vi "PathPlanner_PathConstraints_FromJSON.vi"(11 "JSON String":string) -> (0 "Exists":bool, 3 "PathPlannerConstraints":T1={"MaxVelocityMps;"=0.0, "MaxAccelerationMpsSq;"=0.0, "MaxAngularVelRadPsEc;"=0.0, "MaxAngularAccRadPSecSq"=0.0, "Exists"=FALSE, "Unlimited"=FALSE, "NominalVoltageVolts"=12.0})   [LabVIEW 2019, in "PathPlanner24.lvlib"]
doc: "Create a path constraints object from json string\n \nInputs: \n - JSON String - string - string potentially containing a path constraints definition\n\nOutputs:\n - PathConstraint - cluster - The path constraints defined by the given json\n - Exists - boolean - TRUE if the string contained a path constraints definition"
uses:
  PathPlanner24.lvlib
  TypeDef/PathPlannerPathConstraints.ctl
  <vilib>/Rock Robotics/WPI/ThirdParty/JAS_Junk/TrajLib/Trajectory_Library.lvlib
panel:
  in  "globalConstraints":T2
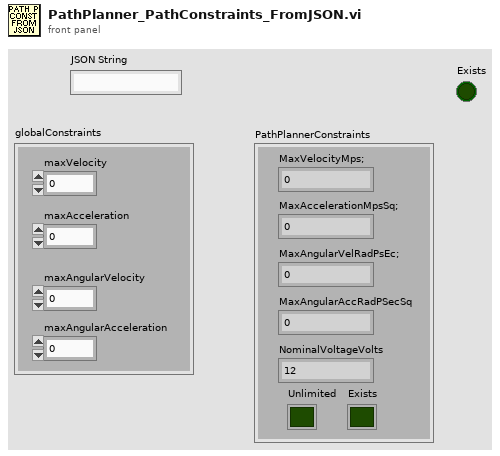
[diagram p1: front panel]
types:
  T1 = typedef "PathPlanner24.lvlib/PathPlannerPathConstraints.ctl" = cluster{"MaxVelocityMps;":dbl, "MaxAccelerationMpsSq;":dbl, "MaxAngularVelRadPsEc;":dbl, "MaxAngularAccRadPSecSq":dbl, "Exists":bool, "Unlimited":bool, "NominalVoltageVolts":dbl}
  T2 = cluster{"maxVelocity":dbl, "maxAcceleration":dbl, "maxAngularVelocity":dbl, "maxAngularAcceleration":dbl}
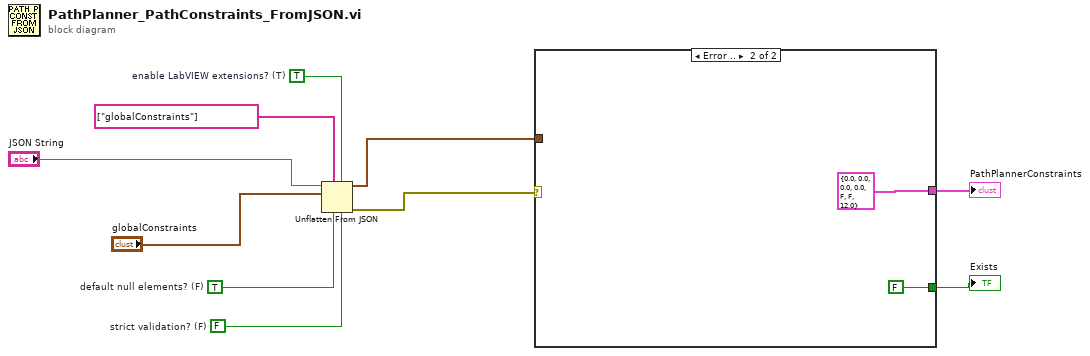
[diagram p0: block diagram]
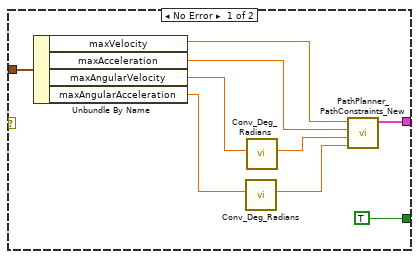
[diagram p2: hidden frame]
diagram:
  w5 = FALSE  # strict validation? (F)
  w6 = TRUE  # default null elements? (F)
  w8 = TRUE  # enable LabVIEW extensions? (T)
  n1 = Unflatten From JSON(path=string[] ["globalConstraints"] ("path 2"), enable LabVIEW extensions? (T)=w8, JSON string="JSON String", type and defaults="globalConstraints", default null elements? (F)=w6, strict validation? (F)=w5) -> (value=w3:T2, error out=w4:errorcluster)  [unwired: 1 in]
  n2 = case shown="Error .." w4 {
    tunnel: w3 -> [w19 _]
    tunnel: [w18 T1 {"MaxVelocityMps;"=0.0, "MaxAccelerationMpsSq;"=0.0, "MaxAngularVelRadPsEc;"=0.0, "MaxAngularAccRadPSecSq"=0.0, "Exists"=FALSE, "Unlimited"=FALSE, "NominalVoltageVolts"=12.0} ("PathPlannerConstraints")] -> w2
    tunnel: [TRUE FALSE] -> w1
    frame No Error {
      n3 = Unbundle By Name(w19) -> ("maxVelocity"=w17:dbl, "maxAcceleration"=w16:dbl, "maxAngularVelocity"=w15:dbl, "maxAngularAcceleration"=w13:dbl)
      n4 = call <vilib>:"Conv_Deg_Radians.vi"("Degress"=w13) -> ("Radians"=w12:dbl)  [unwired: 10 in]
      n5 = call <vilib>:"Conv_Deg_Radians.vi"("Degress"=w15) -> ("Radians"=w14:dbl)  [unwired: 10 in]
      n6 = call "PathPlanner_PathConstraints_New.vi"("MaxAngularAccRadPSecSq"=w12, "MaxAngularVelRadPsEc;"=w14, "MaxAccelerationMpsSq;"=w16, "MaxVelocityMps;"=w17) -> ("PathPlannerConstraints"=w18:T1)  [unwired: 7 in]
    }
    frame Error {
    }
  }
  "PathPlannerConstraints" <- w2
  "Exists" <- w1
